vi "python_node_example.vi"() -> ()   [LabVIEW 2024]
uses:
  <vilib>/Python/Open Anaconda Python Session.vi
panel:
  out "return_tuple":cluster{i32, i32, bool[]}
  out "return_dict":T1
  out "return_tuple_list":cluster{i32, i32, bool[]}[](array[cluster])
  out "return_list":bool[](array[boolean])
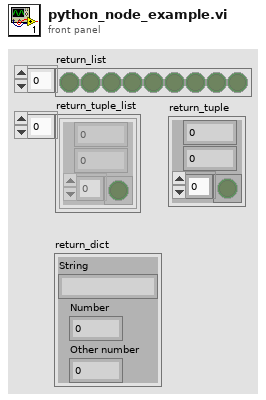
[diagram p1: front panel]
types:
  T1 = cluster{"String":string, "Number":i32, "Other number":i32}
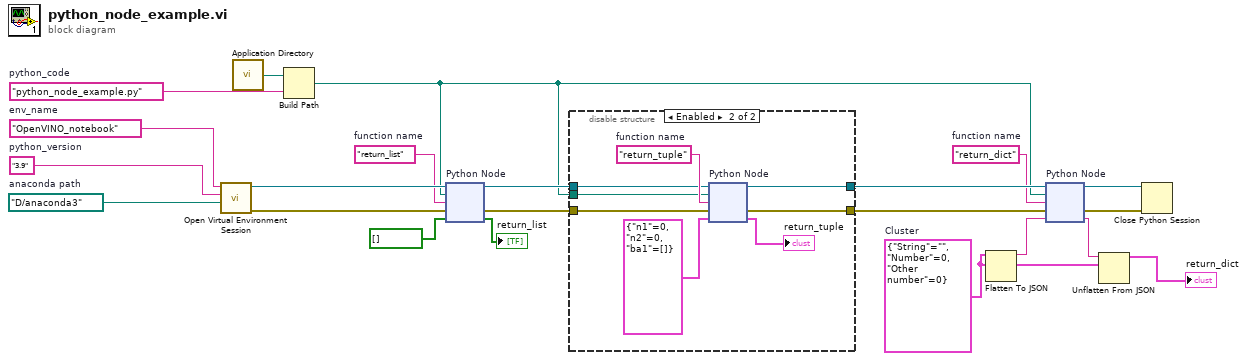
[diagram p0: block diagram]
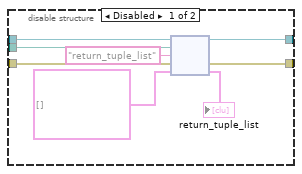
[diagram p2: hidden frame]
diagram:
  w1 = path "D:/anaconda3"  # anaconda path
  w3 = "python_node_example.py"  # python_code
  w5 = "OpenVINO_notebook"  # env_name
  w7 = "return_dict"  # function name
  w9 = T1 {"String"="", "Number"=0, "Other number"=0}  # Cluster
  w20 = "return_list"  # function name
  w6 = "3.9"  # python_version
  n1 = call-poly <vilib>:"Open Virtual Environment Session.vi"("Anaconda path"=w1, "Python version"=w6, "Env name"=w5) -> ("error out"=w21:errorcluster, "session out"=w22:refnum<k35>)  [unwired: 7 in]
  n2 = call <vilib>:"Application Directory.vi"() -> ("Application Directory"=w4:path)
  n3 = Build Path(base path=w4, name or relative path=w3) -> (appended path=w2:path)
  n4 = node "Python Node"(w22, w2, w20, w21, bool[] []) -> (w17:refnum<k35>, w16:errorcluster, →"return_list":bool[])  [unwired: 2 out]
  n5 = disable-structure shown="Enabled" {
    disable-tunnel: w17 -> [w29 w37]
    disable-tunnel: w16 -> [w28 w36]
    disable-tunnel: [w27 w35] -> w15
    disable-tunnel: [w26 w34] -> w14
    disable-tunnel: w2 -> [w23 w33]
    frame Disabled {
      n6 = node(w29, w23, "return_tuple_list" ("function name"), w28, cluster{i32, i32, bool[]}[] []) -> (w27:refnum<k35>, w26:errorcluster, →"return_tuple_list":cluster{i32, i32, bool[]}[])  [unwired: 2 out]
    }
    frame Enabled {
      w38 = "return_tuple"  # function name
      n7 = node "Python Node"(w37, w33, w38, w36, cluster{"n1":i32, "n2":i32, "ba1":bool[]} {"n1"=0, "n2"=0, "ba1"=[]} ("Cluster")) -> (w35:refnum<k35>, w34:errorcluster, →"return_tuple":cluster{"n1":i32, "n2":i32, "ba1":bool[]})  [unwired: 2 out]
    }
  }
  n8 = Flatten To JSON(anything=w9) -> (JSON string=w11:string)  [unwired: 2 in, 1 out]
  n9 = node "Python Node"(w15, w2, w7, w14, w11) -> (w19:refnum<k35>, w18:errorcluster, w10:string)  [unwired: 2 out]
  n10 = Unflatten From JSON(JSON string=w10, type and defaults=w9) -> (value=→"return_dict":T1)  [unwired: 5 in, 1 out]
  n11 = Close Python Session(session in=w19, error in=w18) -> ()  [unwired: 1 out]
